vi "LMB_WallFollow_SetHeading.vi"(8 "Follow Right?":bool=TRUE, 11 "Distance":i32) -> (3 "heading":i32)   [LabVIEW 2012]
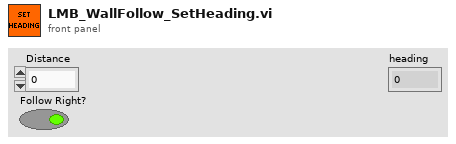
[diagram p1: front panel]
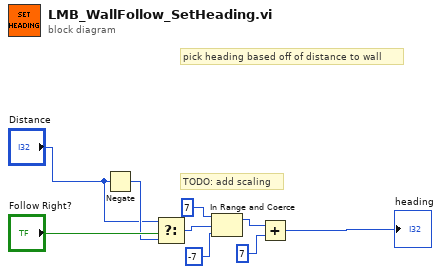
[diagram p0: block diagram]
diagram:
  # "pick heading based off of distance to wall"
  # "TODO: add scaling"
  n1 = Negate(x="Distance") -> (-x=w8:i32)
  n2 = Select(t="Distance", s="Follow Right?", f=w8) -> (s? t:f=w4:i32)
  n3 = In Range and Coerce(upper limit=7, x=w4, lower limit=-7) -> (coerced(x)=w1:i32)  [unwired: 1 out]
  n4 = Add(x=w1, y=7) -> (x+y=→"heading":i32)
